vi "Format when received message logger (SubVI).vi"(1 "received message":string, 2 "queue name":string) -> (0 "info to log":string)   [LabVIEW 2016]
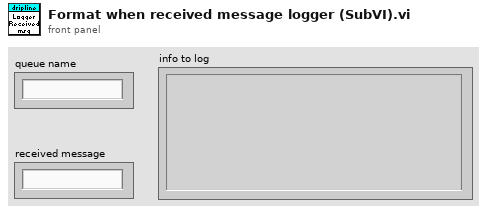
[diagram p1: front panel]
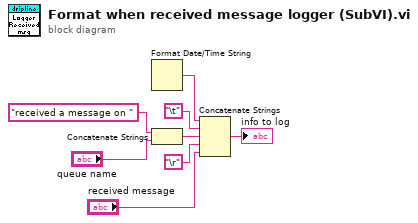
[diagram p0: block diagram]
diagram:
  n1 = Format Date/Time String() -> (date/time string=w4:string)  [unwired: 3 in]
  n2 = Concatenate Strings("received a message on " ("string"), "queue name") -> (w2:string)
  n3 = Concatenate Strings(w4, "\t", w2, "\r", "received message") -> (→"info to log":string)
